vi "QAQC_vacon.vi"() -> ()   [LabVIEW 2015]
uses:
  GlobalPath.vi
  GlobalData.vi
  GlobalVi.vi
panel:
  out "PanelName":string
  in  "ptfe 6":bool caption="Open the vi for the QAQC planarity measurements of the frame+cooling bar region"
  in  "Done with the QAQC?":bool
  in  "ptfe 5":bool caption="Open the vi for the QAQC planarity measurements of the pillar region"
  in  "ptfe 2":bool caption="Check that the table vacuum is ON"
  # "QAQC with vacuum on"
  # "Start QAQC process"
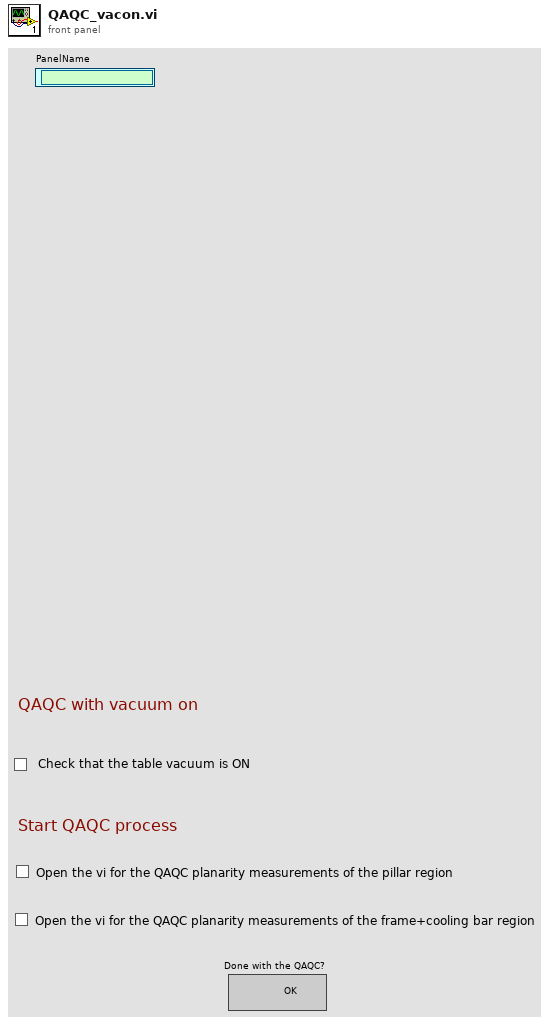
[diagram p1: front panel]
types:
  T1 = enum16{"open", "replace", "create", "open or create", "replace or create", "replace or create with confirmation"}
  T2 = enum32{"Bad", "Idle", "Run top level", "Running"}
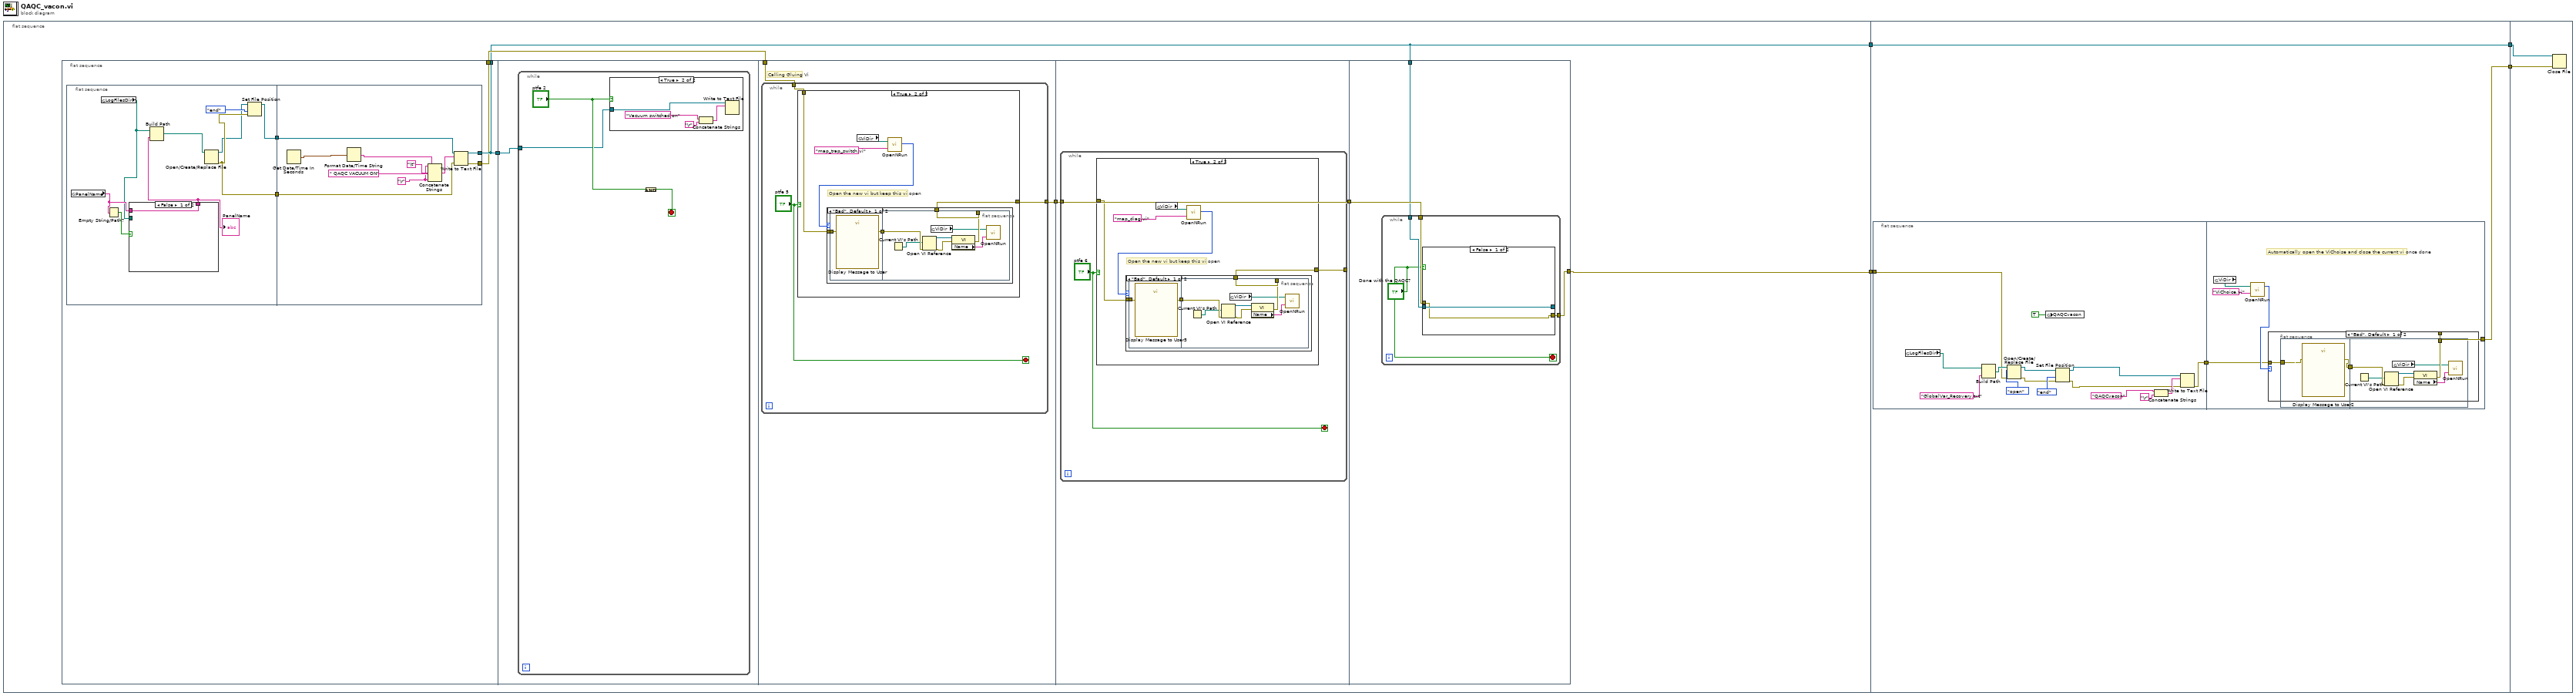
[diagram p0: block diagram]
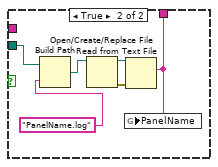
[diagram p2: hidden frame]
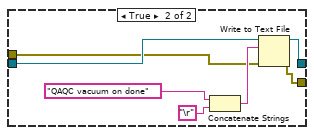
[diagram p8: hidden frame]
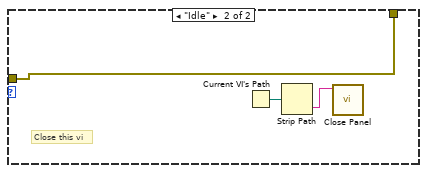
[diagram p9: hidden frame]
diagram:
  n1 = flat-sequence {
    tunnel: [w8] -> w3
    tunnel: [w5] -> w1
    tunnel: [w115] -> w4
    tunnel: w3 -> [w114]
    tunnel: [w114] -> w2
    tunnel: w1 -> [w112]
    tunnel: w4 -> [w152]
    tunnel: w2 -> [w151]
    frame #0 {
      n2 = flat-sequence {
        tunnel: [w13] -> w10
        tunnel: [w13] -> w8
        tunnel: [w12] -> w9
        tunnel: w10 -> [w41]
        tunnel: w9 -> [w50]
        tunnel: [w49] -> w7
        tunnel: w7 -> [w73]
        tunnel: [w73] -> w6
        tunnel: w6 -> [w98]
        tunnel: w8 -> [w97]
        tunnel: [w96] -> w5
        frame #0 {
          n3 = flat-sequence {
            tunnel: [w19] -> w14
            tunnel: [w21] -> w11
            tunnel: w14 -> [w36]
            tunnel: [w35] -> w13
            tunnel: [w34] -> w12
            tunnel: w11 -> [w33]
            frame #0 {
              n4 = global read "GlobalData.vi" "PanelName"() -> (w18:string)
              n5 = global read "GlobalPath.vi" "LogFilesDir"() -> (w15:path)
              n6 = Empty String/Path?(string/path=w18) -> (empty?=w17:bool)
              n7 = case shown="False" w17 {
                tunnel: w15 -> [_ w30]
                tunnel: [w24 w25] -> w16
                tunnel: w18 -> [w24 _]
                frame False {
                }
                frame True {
                  n8 = Build Path(base path=w30, name or relative path="PanelName.log") -> (appended path=w29:path)
                  n9 = Open/Create/Replace File(file path (use dialog)=w29) -> (refnum out=w26:refnum<file>, error out=w27:errorcluster)  [unwired: 5 in, 1 out]
                  n10 = Read from Text File(file (use dialog)=w26, error in=w27) -> (text=w25:string)  [unwired: 2 in, 3 out]
                  n11 = global write "GlobalData.vi" "PanelName"(w25) -> ()
                }
              }
              "PanelName" <- w16
              n12 = Build Path(base path=w15, name or relative path=w16) -> (appended path=w23:path)
              n13 = Open/Create/Replace File(file path (use dialog)=w23) -> (refnum out=w20:refnum<file>, error out=w21:errorcluster)  [unwired: 5 in, 1 out]
              n14 = Set File Position(refnum=w20, from (0:start)=enum16{"start", "end", "current"}."end", error in=w21) -> (refnum out=w19:refnum<file>)  [unwired: 1 in, 1 out]
            }
            frame #1 {
              w31 = "\r"
              n15 = Get Date/Time In Seconds() -> (seconds since 1Jan1904=w32:timestamp)
              n16 = Format Date/Time String(seconds (now)=w32) -> (date/time string=w38:string)  [unwired: 2 in]
              n17 = Concatenate Strings(w31, w38, "\t", " QAQC VACUUM ON", w31) -> (w37:string)
              n18 = Write to Text File(file (use dialog)=w36, text=w37, error in=w33) -> (refnum out=w35:refnum<file>, error out=w34:errorcluster)  [unwired: 1 in, 1 out]
            }
          }
        }
        frame #1 {
          n19 = while {
            tunnel: w41 -> [w42]
            stop <- w44 stop-if-true
            n20 = case shown="True" "ptfe 2" {
              tunnel: w42 -> [_ w45]
              frame False {
              }
              frame True {
                n21 = Concatenate Strings("Vacuum switched on", "\r") -> (w48:string)
                n22 = Write to Text File(file (use dialog)=w45, text=w48) -> ()  [unwired: 2 in, 3 out]
              }
            }
            n23 = Compound Arithmetic op=AND("ptfe 2") -> (w44:bool)
          }
        }
        frame #2 {
          # "Calling Gluing Vi"
          n24 = while {
            tunnel: w50 -> [w53]
            tunnel: [w52] -> w49
            stop <- "ptfe 5" stop-if-true
            n25 = case shown="True" "ptfe 5" {
              tunnel: w53 -> [w54 w56]
              tunnel: [w54 w55] -> w52
              frame False {
              }
              frame True {
                # "Open the new vi but keep this vi open"
                n26 = global read "GlobalPath.vi" "ViDir"() -> (w59:path)
                n27 = call "OpenNRun.vi"("VI name"="map_trap_switch.vi", "ViDirPath"=w59) -> ("Execution:State"=w58:T2)
                n28 = case shown="\"Bad\", Default" w58 {
                  tunnel: [w62 w72] -> w55
                  tunnel: w56 -> [w61 w72]
                  frame "Bad", Default {
                    n29 = flat-sequence {
                      tunnel: w61 -> [w63]
                      tunnel: [w64] -> w60
                      tunnel: [w68] -> w62
                      tunnel: w60 -> [w67]
                      frame #0 {
                        n30 = call "Display Message to User"("error in (no error)"=w63) -> ("error out"=w64:errorcluster)  [unwired: 9 in, 1 out]
                      }
                      frame #1 {
                        n31 = Current VI's Path() -> (path=w65:path)
                        n32 = Open VI Reference(vi path=w65, error in (no error)=w67) -> (vi reference=w71:refnum<vi>, error out=w70:errorcluster)  [unwired: 4 in]
                        n33 = global read "GlobalPath.vi" "ViDir"() -> (w66:path)
                        n34 = property class="VI"(reference=w71, error in=w70) -> (error out=w68:errorcluster, "Name"=w69:string)  [unwired: 1 out]
                        n35 = call "OpenNRun.vi"("VI name"=w69, "ViDirPath"=w66) -> ()  [unwired: 1 out]
                      }
                    }
                  }
                  frame "Idle" {
                    # "Program opened"
                  }
                }
              }
            }
          }
        }
        frame #3 {
          n36 = while {
            tunnel: [w76] -> _
            tunnel: w73 -> [w74]
            stop <- "ptfe 6" stop-if-true
            n37 = case shown="True" "ptfe 6" {
              tunnel: w74 -> [w77 w79]
              tunnel: [w77 w78] -> w76
              frame False {
              }
              frame True {
                # "Open the new vi but keep this vi open"
                n38 = global read "GlobalPath.vi" "ViDir"() -> (w82:path)
                n39 = call "OpenNRun.vi"("VI name"="map_diag.vi", "ViDirPath"=w82) -> ("Execution:State"=w81:T2)
                n40 = case shown="\"Bad\", Default" w81 {
                  tunnel: [w85 w95] -> w78
                  tunnel: w79 -> [w84 w95]
                  frame "Bad", Default {
                    n41 = flat-sequence {
                      tunnel: w84 -> [w86]
                      tunnel: [w87] -> w83
                      tunnel: [w91] -> w85
                      tunnel: w83 -> [w90]
                      frame #0 {
                        n42 = call "Display Message to User3"("error in (no error)"=w86) -> ("error out"=w87:errorcluster)  [unwired: 9 in, 1 out]
                      }
                      frame #1 {
                        n43 = Current VI's Path() -> (path=w88:path)
                        n44 = Open VI Reference(vi path=w88, error in (no error)=w90) -> (vi reference=w94:refnum<vi>, error out=w93:errorcluster)  [unwired: 4 in]
                        n45 = global read "GlobalPath.vi" "ViDir"() -> (w89:path)
                        n46 = property class="VI"(reference=w94, error in=w93) -> (error out=w91:errorcluster, "Name"=w92:string)  [unwired: 1 out]
                        n47 = call "OpenNRun.vi"("VI name"=w92, "ViDirPath"=w89) -> ()  [unwired: 1 out]
                      }
                    }
                  }
                  frame "Idle" {
                    # "Program opened"
                  }
                }
              }
            }
          }
        }
        frame #4 {
          n48 = while {
            tunnel: w98 -> [w102]
            tunnel: w97 -> [w101]
            tunnel: [w100] -> w96
            stop <- "Done with the QAQC?" stop-if-true
            n49 = case shown="False" "Done with the QAQC?" {
              tunnel: w101 -> [w104 w108]
              tunnel: w102 -> [w103 w107]
              tunnel: [w104 w106] -> _
              tunnel: [w103 w105] -> w100
              frame False {
              }
              frame True {
                n50 = Concatenate Strings("QAQC vacuum on done", "\r") -> (w111:string)
                n51 = Write to Text File(file (use dialog)=w108, text=w111, error in=w107) -> (refnum out=w106:refnum<file>, error out=w105:errorcluster)  [unwired: 1 in, 1 out]
              }
            }
          }
        }
      }
    }
    frame #1 {
      n52 = flat-sequence {
        tunnel: [w119] -> w113
        tunnel: w112 -> [w118]
        tunnel: [w132] -> w115
        tunnel: w113 -> [w131]
        frame #0 {
          n53 = global read "GlobalPath.vi" "LogFilesDir"() -> (w116:path)
          n54 = Build Path(base path=w116, name or relative path="GlobalVar_Recovery.txt") -> (appended path=w128:path)
          n55 = Open/Create/Replace File(file path (use dialog)=w128, error in=w118, operation (0:open)=T1."open") -> (refnum out=w124:refnum<file>, error out=w125:errorcluster)  [unwired: 3 in, 1 out]
          n56 = global write "GlobalVi.vi" "QAQCvacon"(TRUE) -> ()
          n57 = Set File Position(refnum=w124, from (0:start)=enum16{"start", "end", "current"}."end", error in=w125) -> (refnum out=w121:refnum<file>, error out=w120:errorcluster)  [unwired: 1 in]
          n58 = Concatenate Strings("QAQCvacon", "\r") -> (w123:string)
          n59 = Write to Text File(file (use dialog)=w121, text=w123, error in=w120) -> (error out=w119:errorcluster)  [unwired: 1 in, 2 out]
        }
        frame #1 {
          # "Automatically open the ViChoise and close the current vi once done"
          n60 = global read "GlobalPath.vi" "ViDir"() -> (w135:path)
          n61 = call "OpenNRun.vi"("VI name"="ViChoice.vi", "ViDirPath"=w135) -> ("Execution:State"=w134:T2)
          n62 = case shown="\"Bad\", Default" w134 {
            tunnel: [w138 w150] -> w132
            tunnel: w131 -> [w137 w150]
            frame "Bad", Default {
              n63 = flat-sequence {
                tunnel: w137 -> [w140]
                tunnel: [w139] -> w136
                tunnel: [w144] -> w138
                tunnel: w136 -> [w143]
                frame #0 {
                  n64 = call "Display Message to User2"("error in (no error)"=w140) -> ("error out"=w139:errorcluster)  [unwired: 9 in, 1 out]
                }
                frame #1 {
                  n65 = Current VI's Path() -> (path=w141:path)
                  n66 = Open VI Reference(vi path=w141, error in (no error)=w143) -> (vi reference=w147:refnum<vi>, error out=w146:errorcluster)  [unwired: 4 in]
                  n67 = global read "GlobalPath.vi" "ViDir"() -> (w142:path)
                  n68 = property class="VI"(reference=w147, error in=w146) -> (error out=w144:errorcluster, "Name"=w145:string)  [unwired: 1 out]
                  n69 = call "OpenNRun.vi"("VI name"=w145, "ViDirPath"=w142) -> ()  [unwired: 1 out]
                }
              }
            }
            frame "Idle" {
              # "Close this vi"
              n70 = Current VI's Path() -> (path=w149:path)
              n71 = Strip Path(path=w149) -> (name=w148:string)  [unwired: 1 out]
              n72 = call <vilib>:"Close Panel.vi"("VI name"=w148) -> ()  [unwired: 10 in, 1 out]
            }
          }
        }
      }
    }
    frame #2 {
      n73 = Close File(refnum=w151, error in=w152) -> ()  [unwired: 2 out]
    }
  }
